vi "Button Size Write.vi"(4 "error in (no error)":errorcluster, 5 "Value":i32, 6 "Container State":T3, 7 "Display State In":T1={"Buttons Displayed"=0, "Button States"=[], "Button Size"=0, "Button Style"=enum."Classic", "Active Button"=0, "Force Regen?"=FALSE, "Tip String Ref"=refnum}) -> (0 "error out":errorcluster, 3 "Display State Out":T1={"Buttons Displayed"=0, "Button States"=[], "Button Size"=0, "Button Style"=enum."Classic", "Active Button"=0, "Force Regen?"=FALSE, "Tip String Ref"=refnum})   [LabVIEW 2018, in "Toolbar.xctl"]
doc: "Set the current toolbar button size."
uses:
  Toolbar.xctl
  <vilib>/_xctls/Container State.ctl
  <vilib>/_xctls/XControlSupport.lvlib
  Toolbar State.ctl
  Button_Class/Button.lvclass
  Button_Class/Type Defs/Button Style.ctl
panel:
  # "Replace the Value Control below with a Control of desired type.\nDo not remove this Control or the others from the connector pane.\nDo not change the connector pane pattern.\nThe Value control should always be the third terminal from top on the input side in the connector pane."
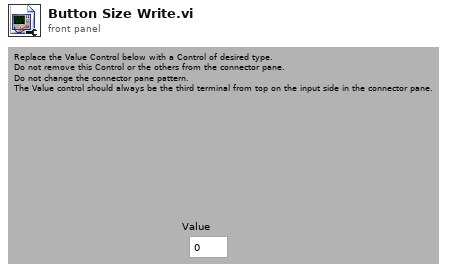
[diagram p1: front panel]
types:
  T1 = typedef "Toolbar.xctl/Toolbar State.ctl" = cluster{"Buttons Displayed":i32, "Button States":refnum<class "Button.lvclass">[], "Button Size":i32, "Button Style":T2, "Active Button":i32, "Force Regen?":bool, "Tip String Ref":refnum<vi>}
  T2 = typedef "Button.lvclass/Button Style.ctl" = enum16{"System", "Modern", "Classic", "Rounded", "Silver", "Ni Theme", "Metallic"}
  T3 = typedef "XControlSupport.lvlib/Container State.ctl" = cluster{"Indicator?":bool, "Run Mode?":bool, " Refnum":refnum<vi>}
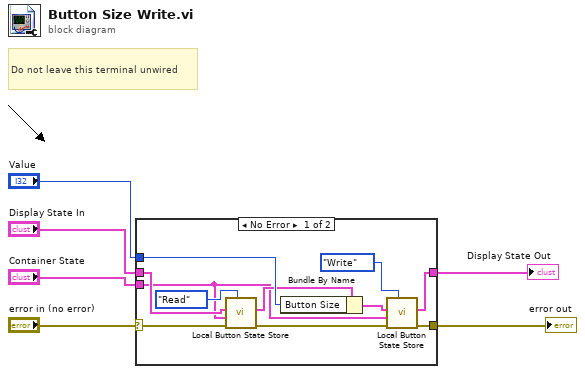
[diagram p0: block diagram]
diagram:
  # "Do not leave this terminal unwired"
  n1 = case shown="No Error" "error in (no error)" {
    selector: "error in (no error)" -> [w9 w18]
    tunnel: [w8 w18] -> w5
    tunnel: "Display State In" -> [w16 w19]
    tunnel: "Value" -> [w17 _]
    tunnel: [w12 w19] -> w2
    tunnel: "Container State" -> [w7 _]
    frame No Error {
      n2 = call "Local Button State Store.vi"("Operation"=enum16{"Read", "Write"}."Read", "error in (no error)"=w9, "Container State"=w7, "Display State In"=w16) -> ("error out"=w10:errorcluster, "Display State Out"=w15:T1)  [unwired: 6 out]
      n3 = Bundle By Name(cluster=w15, "Button Size"=w17) -> (w13:T1)
      n4 = call "Local Button State Store.vi"("Operation"=enum16{"Read", "Write"}."Write", "error in (no error)"=w10, "Container State"=w7, "Display State In"=w13) -> ("error out"=w8:errorcluster, "Display State Out"=w12:T1)  [unwired: 6 out]
    }
    frame Error {
    }
  }
  "error out" <- w5
  "Display State Out" <- w2
